vi "Write U8.vi"(10 "U8":u8, 11 "Event in":refnum<class "Event U8.lvclass">) -> (3 "Event out":refnum<class "Event U8.lvclass">)   [LabVIEW 2016, in "Event Source.lvlib" / "Event U8.lvclass"]
uses:
  Event U8.lvclass
  Event U8.lvclass/Event U8.ctl
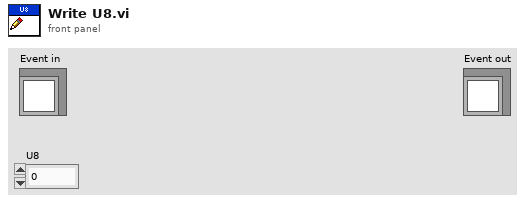
[diagram p1: front panel]
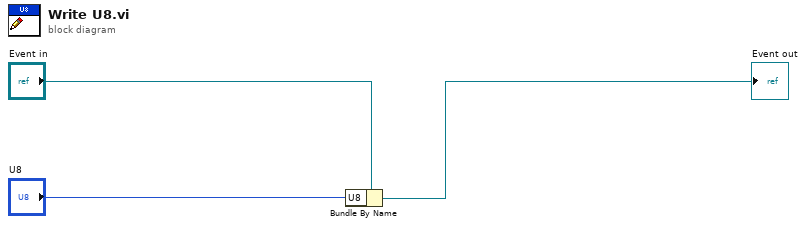
[diagram p0: block diagram]
diagram:
  n1 = Bundle By Name(cluster="Event in", "U8"="U8") -> (→"Event out":refnum<class "Event U8.lvclass">)
